vi "Meas Generate Freq List.vi"(2 "freq. id":i32, 3 "meas setup":T4={"swp cfg"={"N"=0, "R"=0, "f list"=[], "smpl delay"=0.0, "set delay"=0.0, "set delay np"=0.0, "meas root"=path "", "meas name"="", "meas a-index"=FALSE, "rnd sweep"=FALSE, "mode"=enum."Frequency", "swp mode"=enum."Linear", "avg"=0, "subrec"=0, "multi-freq"=FALSE}, "bridge"={"type"=enum."TWM client", "TWM"={"pipe name"="", "parameters"=[], "handle"=0, "fixed aper [s]"=0.0, "f-list [Hz]"=[], "discrete f-list"=FALSE, "unc mode"=enum."None", "unc mcc"=0, "unc first"=FALSE}, "last f"=0.0, "bias comp"={"bias type"=enum."dummy", "VISA"="", "Enable"=FALSE, "channel qu"=[], "channel Uinit"=[]}, "sim mode"=enum."Generic RLC network", "channel idns"=[], "sim phases"=1}, "src"={"type"=enum."Tektronix AFG3101C", "afg"={"VISA"="", "const"=0.0, "gen DC"=FALSE, "ext ref"=FALSE}, "cDAQ dds"={"device"="", "channels"=[], "mclk source"="", "mclk [Hz]"=0.0, "use ext mclk"=FALSE, "fs [Hz]"=0.0, "block [s]"=0.0, "buf [s]"=0.0, "task"="", "cmd queue"=refnum, "proc ref"=refnum, "smpl clock out"="/cDAQ3/PFI0", "export smpl clock"=FALSE, "DC ofs [V]"=[]}, "gain [V/A]"=1.0, "F5xxx session"={"VISA"="", "mode"=enum."AC voltage", "Earth on"=FALSE, "Ext ref lock"=FALSE}}, "results"=refnum} {"src"."cDAQ dds"."channels" min=0 step=1; "bridge"."TWM"."f-list [Hz]" format="%#_6p"; "swp cfg"."f list"."bias" format="%#_3p"; "swp cfg"."f list"."level" format="%#_3p"; "swp cfg"."f list"."fs [Hz]" format="%#_5p"; "swp cfg"."f list"."time [s]" format="%#_3p"; "swp cfg"."f list"."f/fs" format="%#_3p"; "swp cfg"."f list"."periods" format="%#_3f"; "swp cfg"."f list"."f [Hz]" format="%#_5p"}, 4 "config":T1={"swp type"=enum."Frequency", "freq sgl"=1000.0, "swp min"=0.0, "swp max"=0.0, "swp step"=0.0, "swp mode"=enum."Linear", "swp steps"=0, "round abs"=0.0, "round rel"=0.0, "f0 coherent"=FALSE, "min fs"=0.0, "min fs ratio"=0.0, "t int [s]"=0.0, "nper [-]"=0.0, "level sgl"=1000.0, "bias sgl"=1000.0, "single"=FALSE, "sweep"=FALSE, "custom"=FALSE, "swp list"=[], "skip mains"=FALSE, "N base"=0, "N max"=0, "N factor"=0.0, "N variable"=FALSE, "multi-freq"=FALSE} {"bias sgl" format="%#_6p"; "level sgl" format="%#_6p"; "freq sgl" format="%#_6p"}) -> (0 "freq lst":dbl[](array[numeric]) caption="Frequency list [Hz]" format="%#_6p", 1 "flist":T6[](array[typedef]) caption="Sweep list items" {"bias" format="%#_3p"; "level" format="%#_3p"; "fs [Hz]" format="%#_5p"; "time [s]" format="%#_3p"; "f/fs" format="%#_3p"; "periods" format="%#_3f"; "f [Hz]" format="%#_5p"})   [LabVIEW 2013]
doc: "Generate sweep list."
uses:
  Meas Freq Info.ctl
  meas session.ctl
  Meas Sweep Config.ctl
  meas_swp_mode.ctl
  meas_sweep_flist_mode.ctl
  bridge/Bridge Session.ctl
  bridge/Bridge Type.ctl
  drivers/TWM client/TWM Session.ctl
  drivers/TWM client/TWM parameters.ctl
  drivers/TWM client/Meas Proc QWTB Uncertainty Mode.ctl
  bridge/Bridge Bias Session.ctl
  bridge/Bridge Bias Type.ctl
  bridge/Bridge Sim Mode.ctl
  source/Source Session.ctl
  source/Source Type.ctl
  drivers/AFG3101C/AFG3101C Session.ctl
  drivers/cDAQ DDS/cDAQ DDS Session.ctl
  drivers/cDAQ DDS/cDAQ DDS Setup.ctl
  drivers/Fluke 5XXX/top_lev/F5xxx_session.ctl
  drivers/Fluke 5XXX/top_lev/F5xxx_output_mode.ctl
  Meas Results Ref.ctl
  Meas Results.ctl
  bridge/Bridge Frequency Readings Data.ctl
  drivers/TWM client/Meas Proc QWTB Spectrum Data.ctl
  drivers/TWM client/TWM Phase Info.ctl
  Meas Sweep List Generator Config.ctl
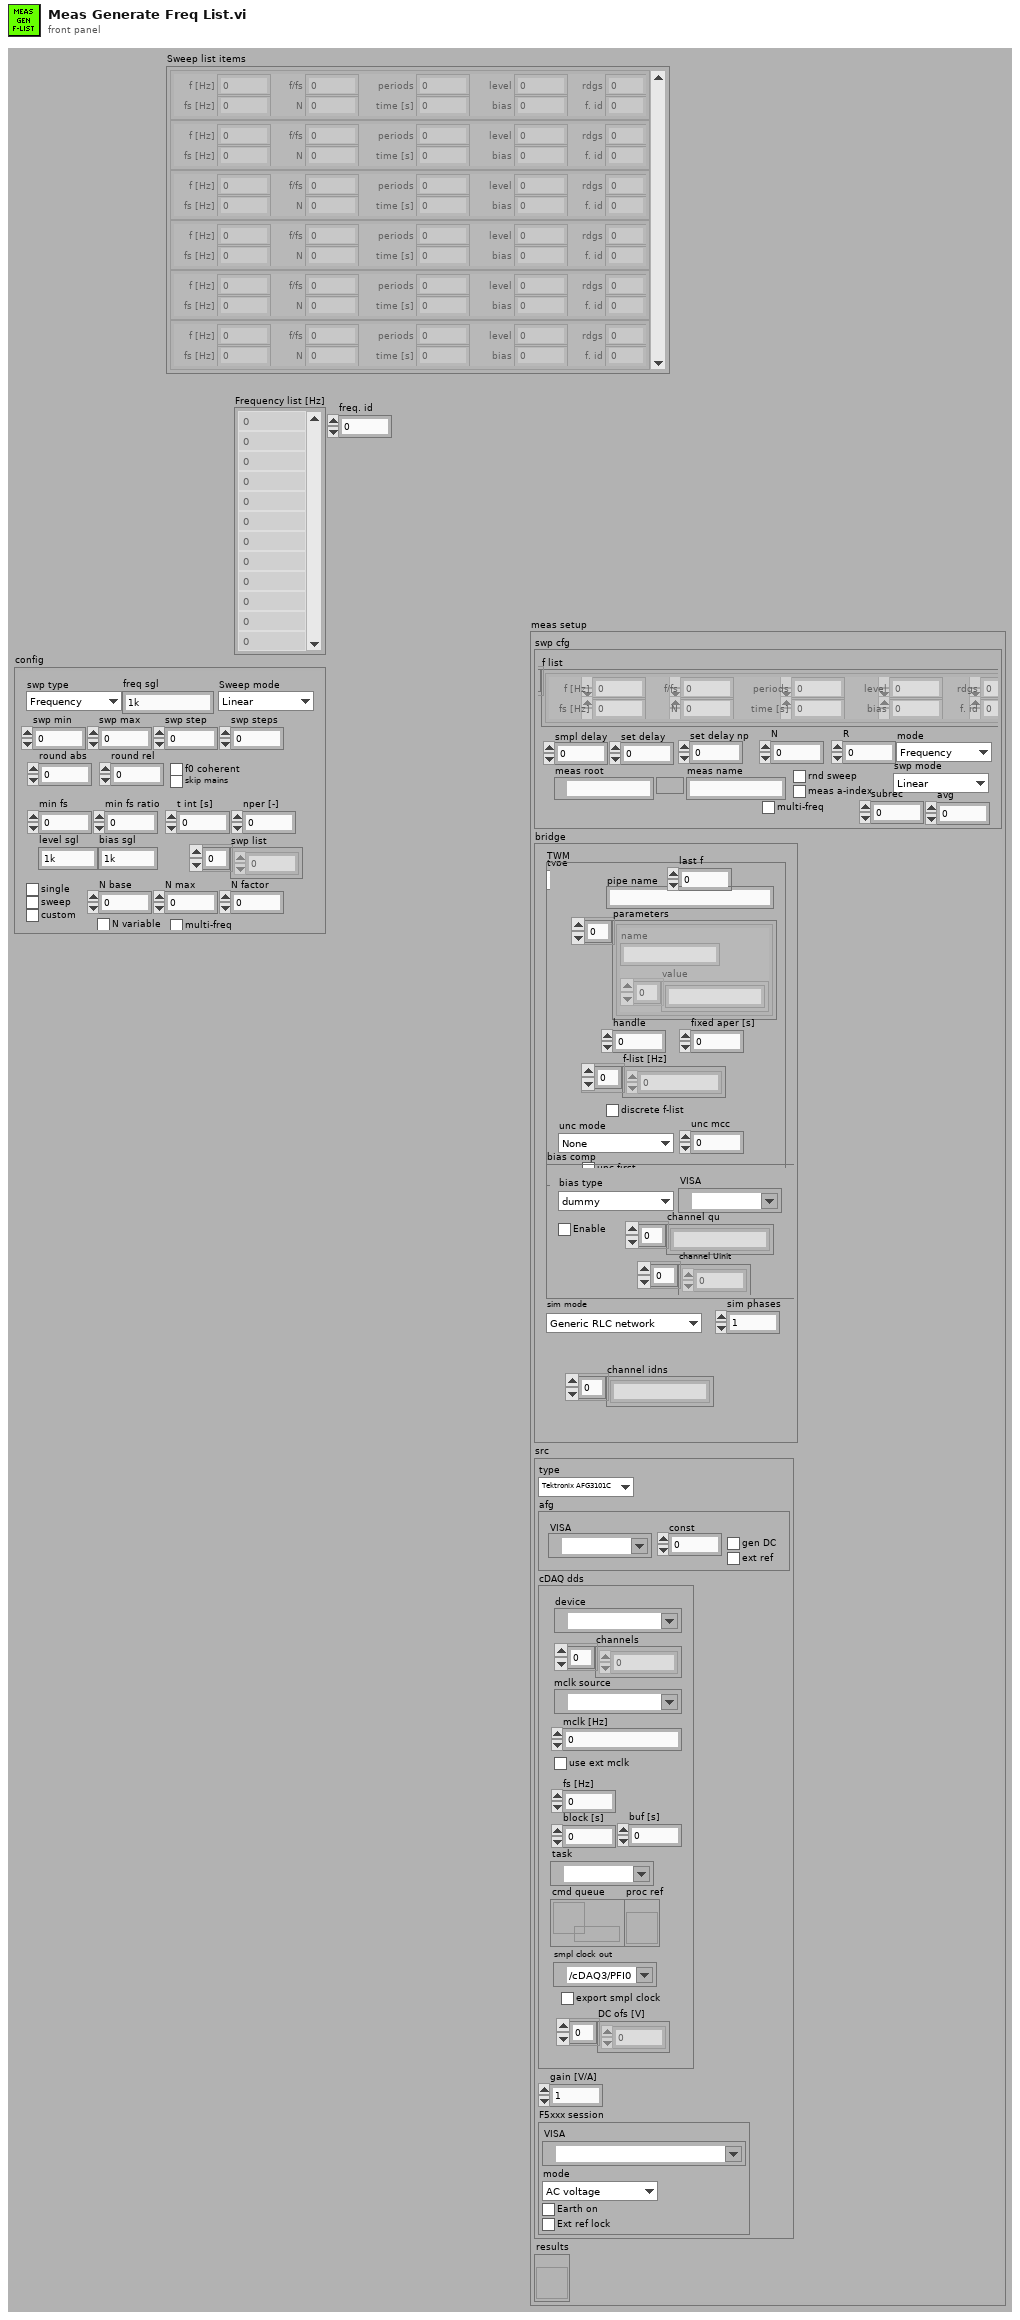
[diagram p1: front panel]
types:
  T1 = typedef "Meas Sweep List Generator Config.ctl" = cluster{"swp type":T2, "freq sgl":dbl, "swp min":dbl, "swp max":dbl, "swp step":dbl, "swp mode":T3, "swp steps":i32, "round abs":dbl, "round rel":dbl, "f0 coherent":bool, "min fs":dbl, "min fs ratio":dbl, "t int [s]":dbl, "nper [-]":dbl, "level sgl":dbl, "bias sgl":dbl, "single":bool, "sweep":bool, "custom":bool, "swp list":dbl[], "skip mains":bool, "N base":i32, "N max":i32, "N factor":dbl, "N variable":bool, "multi-freq":bool}
  T2 = typedef "meas_swp_mode.ctl" = enum16{"Frequency", "Level", "Bias"}
  T3 = typedef "meas_sweep_flist_mode.ctl" = enum16{"Linear", "Log10"}
  T4 = typedef "meas session.ctl" = cluster{"swp cfg":T5, "bridge":T7, "src":T15, "results":T21}
  T5 = typedef "Meas Sweep Config.ctl" = cluster{"N":i32, "R":i32, "f list":T6[], "smpl delay":dbl, "set delay":dbl, "set delay np":dbl, "meas root":path, "meas name":string, "meas a-index":bool, "rnd sweep":bool, "mode":T2, "swp mode":T3, "avg":i32, "subrec":i32, "multi-freq":bool}
  T6 = typedef "Meas Freq Info.ctl" = cluster{"f [Hz]":dbl, "periods":dbl, "f/fs":dbl, "time [s]":dbl, "fs [Hz]":dbl, "N":i32, "level":dbl, "bias":dbl, "rdgs":i32, "f. id":i32}
  T7 = typedef "Bridge Session.ctl" = cluster{"type":T8, "TWM":T9, "last f":dbl, "bias comp":T12, "sim mode":T14, "channel idns":string[], "sim phases":i32}
  T8 = typedef "Bridge Type.ctl" = enum16{"TWM client", "dummy"}
  T9 = typedef "TWM Session.ctl" = cluster{"pipe name":string, "parameters":T10[], "handle":i32, "fixed aper [s]":dbl, "f-list [Hz]":dbl[], "discrete f-list":bool, "unc mode":T11, "unc mcc":i32, "unc first":bool}
  T10 = typedef "TWM parameters.ctl" = cluster{"name":string, "value":string[]}
  T11 = typedef "Meas Proc QWTB Uncertainty Mode.ctl" = enum16{"None", "GUF", "Monte Carlo"}
  T12 = typedef "Bridge Bias Session.ctl" = cluster{"bias type":T13, "VISA":refnum<visa-resource-name>, "Enable":bool, "channel qu":string[], "channel Uinit":dbl[]}
  T13 = typedef "Bridge Bias Type.ctl" = enum16{"dummy", "CMI LiBbias V1.0"}
  T14 = typedef "Bridge Sim Mode.ctl" = enum16{"Generic RLC network", "Interchannel transfer"}
  T15 = typedef "Source Session.ctl" = cluster{"type":T16, "afg":T17, "cDAQ dds":T18, "gain [V/A]":dbl, "F5xxx session":T19}
  T16 = typedef "Source Type.ctl" = enum16{"Tektronix AFG3101C", "cDAQ DAC", "Fluke 5xxx", "Agilent 33120A", "dummy"}
  T17 = typedef "AFG3101C Session.ctl" = cluster{"VISA":refnum<visa-resource-name>, "const":dbl, "gen DC":bool, "ext ref":bool}
  T18 = typedef "cDAQ DDS Session.ctl" = cluster{"device":tag, "channels":i32[], "mclk source":tag, "mclk [Hz]":dbl, "use ext mclk":bool, "fs [Hz]":dbl, "block [s]":dbl, "buf [s]":dbl, "task":refnum<k21>, "cmd queue":refnum<queue>, "proc ref":refnum<vi>, "smpl clock out":tag, "export smpl clock":bool, "DC ofs [V]":dbl[]}
  T19 = typedef "F5xxx_session.ctl" = cluster{"VISA":refnum<visa-resource-name>, "mode":T20, "Earth on":bool, "Ext ref lock":bool}
  T20 = typedef "F5xxx_output_mode.ctl" = enum16{"AC voltage", "AC current"}
  T21 = typedef "Meas Results Ref.ctl" = refnum<vi>
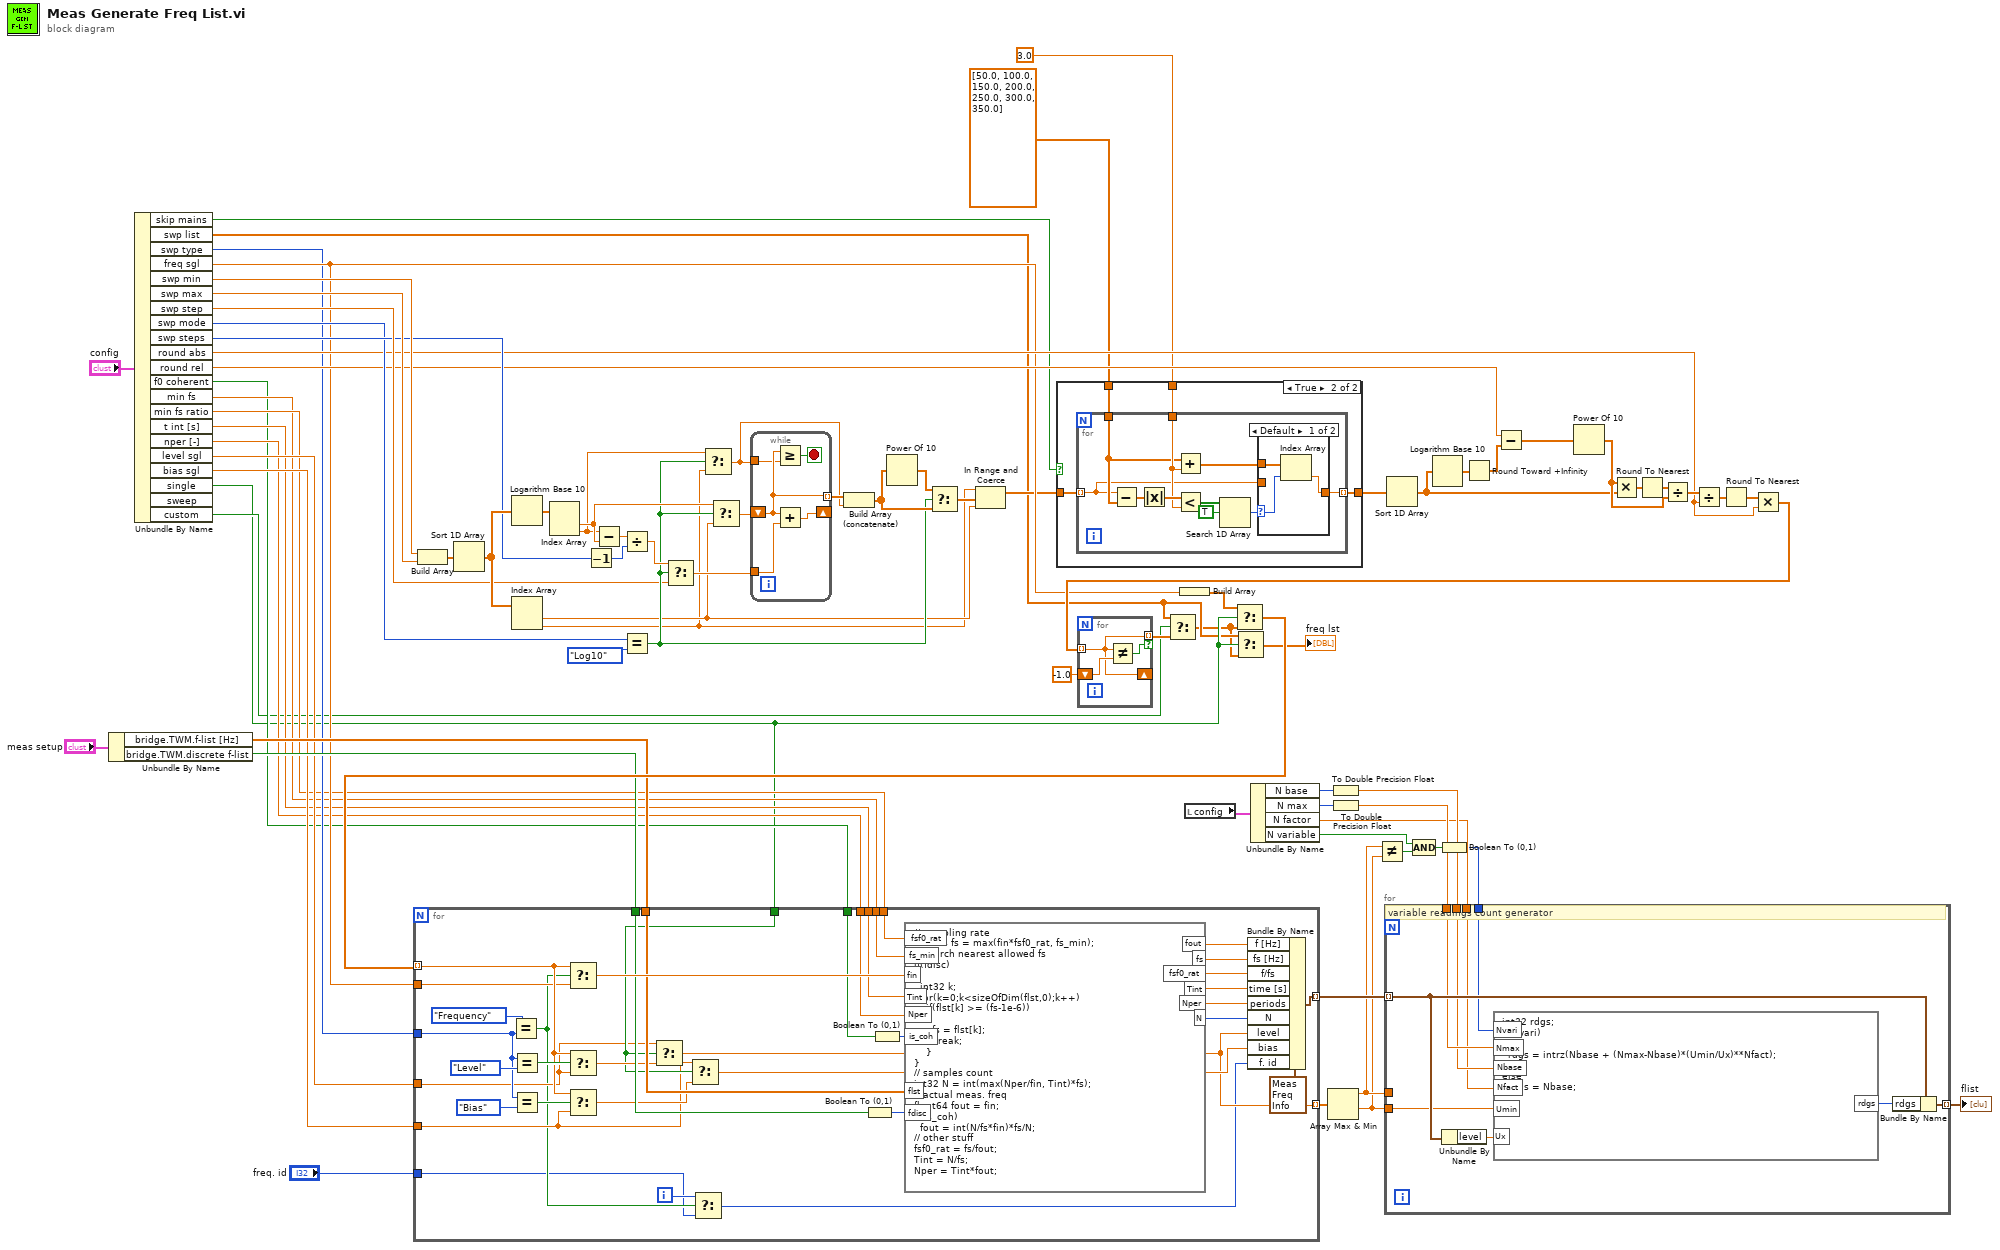
[diagram p0: block diagram]
diagram:
  n1 = Unbundle By Name("meas setup") -> ("bridge.TWM.f-list [Hz]"=w45:dbl[], "bridge.TWM.discrete f-list"=w46:bool)
  n2 = Unbundle By Name("config") -> ("skip mains"=w21:bool, "swp list"=w2:dbl[], "swp type"=w35:T2, "freq sgl"=w36:dbl, "swp min"=w43:dbl, "swp max"=w42:dbl, "swp step"=w41:dbl, "swp mode"=w39:T3, "swp steps"=w40:i32, "round abs"=w37:dbl, "round rel"=w38:dbl, "f0 coherent"=w28:bool, "min fs"=w31:dbl, "min fs ratio"=w32:dbl, "t int [s]"=w30:dbl, "nper [-]"=w29:dbl, "level sgl"=w34:dbl, "bias sgl"=w33:dbl, "single"=w4:bool, "custom"=w27:bool)  [unwired: 1 out]
  n3 = Build Array(w43, w42) -> (w80:dbl[])
  n4 = Sort 1D Array(array=w80) -> (sorted array=w79:dbl[])
  n5 = Logarithm Base 10(1:w79) -> (0:w78:dbl[])
  n6 = Index Array(array=w79) -> (element #1=w48:dbl, element #2=w47:dbl)  [unwired: 2 in]
  n7 = Index Array(array=w78) -> (element #1=w75:dbl, element #2=w73:dbl)  [unwired: 2 in]
  n8 = Decrement(x=w40) -> (x-1=w50:i32)
  n9 = Subtract(x=w73, y=w75) -> (x-y=w77:dbl)
  n10 = Divide(x=w77, y=w50) -> (x/y=w76:dbl)
  n11 = Equal?(x=w39, y=meas_sweep_flist_mode."Log10") -> (x = y?=w65:bool)
  n12 = Select(t=w76, s=w65, f=w41) -> (s? t:f=w74:dbl)
  n13 = Select(t=w73, s=w65, f=w47) -> (s? t:f=w68:dbl)
  n14 = Select(t=w75, s=w65, f=w48) -> (s? t:f=w71:dbl)
  n15 = while {
    tunnel: w74 -> [w85]
    tunnel: w68 -> [w82]
    shift-right: [w84] -> _
    shift-left: w71 -> [w83]
    tunnel: [w83] -> w72 mode=indexing
    stop <- w81 stop-if-true
    n16 = Greater Or Equal?(x=w83, y=w82) -> (x >= y?=w81:bool)
    n17 = Add(x=w83, y=w85) -> (x+y=w84:dbl)
  }
  n18 = Build Array (concatenate)(w72, w68) -> (w69:dbl[])
  n19 = Power Of 10(x=w69) -> (10^x=w70:dbl[])
  n20 = Select(t=w70, s=w65, f=w69) -> (s? t:f=w49:dbl[])
  n21 = In Range and Coerce(upper limit=w47, x=w49, lower limit=w48) -> (coerced(x)=w25:dbl[])  [unwired: 1 out]
  n22 = case shown="True" w21 {
    tunnel: w25 -> [w86 w90]
    tunnel: [w86 w89] -> w24
    tunnel: dbl[] [50.0, 100.0, 150.0, 200.0, 250.0, 300.0, 350.0] -> [_ w88]
    tunnel: 3.0 -> [_ w87]
    frame False {
    }
    frame True {
      n23 = for {
        tunnel: w90 -> [w92] mode=indexing
        tunnel: [w93] -> w89 mode=indexing
        tunnel: w88 -> [w97]
        tunnel: w87 -> [w98]
        n24 = Subtract(x=w92, y=w97) -> (x-y=w100:dbl[])
        n25 = Absolute Value(x=w100) -> (abs(x)=w99:dbl[])
        n26 = Add(x=w97, y=w98) -> (x+y=w91:dbl[])
        n27 = Less?(x=w99, y=w98) -> (x < y?=w96:bool[])
        n28 = Search 1D Array(1D array=w96, element=TRUE) -> (index of element=w94:i32)  [unwired: 1 in]
        n29 = case shown="Default" w94 {
          selector: w94 -> [w102 _]
          tunnel: [w101 w104] -> w93
          tunnel: w92 -> [_ w104]
          tunnel: w91 -> [w103 _]
          frame Default {
            n30 = Index Array(array=w103, index=w102) -> (element=w101:dbl)
          }
          frame -1 {
          }
        }
      }
    }
  }
  n31 = Build Array(w36) -> (w52:dbl[])
  n32 = local read "config"() -> (w19:T1)
  n33 = Unbundle By Name(w19) -> ("N base"=w16:i32, "N max"=w13:i32, "N factor"=w12:dbl, "N variable"=w7:bool)
  n34 = To Double Precision Float(number=w16) -> (double precision float=w15:dbl)
  n35 = To Double Precision Float(number=w13) -> (double precision float=w17:dbl)
  n36 = Sort 1D Array(array=w24) -> (sorted array=w58:dbl[])
  n37 = Logarithm Base 10(1:w58) -> (0:w64:dbl[])
  n38 = Round Toward +Infinity(x=w64) -> (ceil(x): smallest int >= x=w63:dbl[])
  n39 = Subtract(x=w38, y=w63) -> (x-y=w62:dbl[])
  n40 = Power Of 10(x=w62) -> (10^x=w59:dbl[])
  n41 = Multiply(x=w59, y=w58) -> (x*y=w61:dbl[])
  n42 = Round To Nearest(number=w61) -> (nearest integer value=w60:dbl[])
  n43 = Divide(x=w60, y=w59) -> (x/y=w57:dbl[])
  n44 = Divide(x=w57, y=w37) -> (x/y=w56:dbl[])
  n45 = Round To Nearest(number=w56) -> (nearest integer value=w55:dbl[])
  n46 = Multiply(x=w55, y=w37) -> (x*y=w54:dbl[])
  n47 = for {
    tunnel: w54 -> [w106] mode=indexing
    shift-right: [w106] -> _
    shift-left: -1.0 -> [w107]
    tunnel: [w106] -> w53 mode=indexing if=w105
    n48 = Not Equal?(x=w106, y=w107) -> (x != y?=w105:bool)
  }
  n49 = Select(t=w2, s=w27, f=w53) -> (s? t:f=w1:dbl[])
  n50 = Select(t=w52, s=w4, f=w1) -> (s? t:f=w51:dbl[])
  n51 = for {
    tunnel: w51 -> [w137] mode=indexing
    tunnel: [w143] -> w20 mode=indexing
    tunnel: w46 -> [w126]
    tunnel: w45 -> [w127]
    tunnel: w4 -> [w122]
    tunnel: w36 -> [w121]
    tunnel: w35 -> [w120]
    tunnel: w34 -> [w119]
    tunnel: w33 -> [w118]
    tunnel: w32 -> [w117]
    tunnel: w31 -> [w116]
    tunnel: w30 -> [w115]
    tunnel: w29 -> [w114]
    tunnel: w28 -> [w113]
    tunnel: [w112] -> w18 mode=indexing
    tunnel: "freq. id" -> [w108]
    i -> [w110]
    n52 = Equal?(x=meas_swp_mode."Frequency", y=w120) -> (x = y?=w111:bool)
    n53 = Equal?(x=w120, y=meas_swp_mode."Level") -> (x = y?=w140:bool)
    n54 = Equal?(x=w120, y=meas_swp_mode."Bias") -> (x = y?=w139:bool)
    n55 = Select(t=w137, s=w111, f=w121) -> (s? t:f=w136:dbl)
    n56 = Select(t=w137, s=w140, f=w119) -> (s? t:f=w125:dbl)
    n57 = Select(t=w137, s=w139, f=w118) -> (s? t:f=w124:dbl)
    n58 = Select(t=w119, s=w122, f=w125) -> (s? t:f=w112:dbl)
    n59 = Select(t=w118, s=w122, f=w124) -> (s? t:f=w123:dbl)
    n60 = Select(t=w110, s=w111, f=w108) -> (s? t:f=w109:i32)
    n61 = Boolean To (0,1)(Boolean=w126) -> (0, 1=w128:i16)
    n62 = Boolean To (0,1)(Boolean=w113) -> (0, 1=w135:i16)
    n63 = formula code="// sampling rate\nfloat64 fs = max(fin*fsf0_rat, fs_min);\n// search nearest allowed fs\nif(fdisc)\n{\n  int32 k;\n  for(k=0;k<sizeOfDim(flst,0);k++)\n    if(flst[k] >= (fs-1e-6))\n    {\n      fs = flst[k];\n      break;\n    }\n}\n// samples count\nint32 N = int(max(Nper/fin, Tint)*fs);\n// actual meas. freq\nfloat64 fout = fin;\nif(is_coh)\n  fout = int(N/fs*fin)*fs/N;\n// other stuff\nfsf0_rat = fs/fout;\nTint = N/fs;\nNper = Tint*fout;"("fsf0_rat"=w117, "fs_min"=w116, "Tint"=w115, "Nper"=w114, "fin"=w136, "is_coh"=w135, "flst"=w127, "fdisc"=w128) -> ("fout"=w134:dbl, "fs"=w133:dbl, "Tint"=w131:dbl, "Nper"=w130:dbl, "fsf0_rat"=w132:dbl, "N"=w129:i32)
    n64 = Bundle By Name(cluster=T6 {"f [Hz]"=0.0, "periods"=0.0, "f/fs"=0.0, "time [s]"=0.0, "fs [Hz]"=0.0, "N"=0, "level"=0.0, "bias"=0.0, "rdgs"=0, "f. id"=0} ("Cluster"), "f [Hz]"=w134, "fs [Hz]"=w133, "f/fs"=w132, "time [s]"=w131, "periods"=w130, "N"=w129, "level"=w112, "bias"=w123, "f. id"=w109) -> (w143:T6)
  }
  n65 = Select(t=w2, s=w4, f=w1) -> (s? t:f=→"freq lst":dbl[])
  n66 = Array Max & Min(array=w18) -> (max value=w10:dbl, min value=w9:dbl)  [unwired: 2 out]
  n67 = Not Equal?(x=w10, y=w9) -> (x != y?=w8:bool)
  n68 = Compound Arithmetic op=AND(w7, w8) -> (w6:bool)
  n69 = Boolean To (0,1)(Boolean=w6) -> (0, 1=w11:i16)
  n70 = for {
    tunnel: w20 -> [w153] mode=indexing
    tunnel: w9 -> [w151]
    tunnel: w10 -> [_]
    tunnel: w17 -> [w150]
    tunnel: w15 -> [w149]
    tunnel: [w152] -> w14 mode=indexing
    tunnel: w12 -> [w148]
    tunnel: w11 -> [w146]
    # "variable readings count generator"
    n71 = Unbundle By Name(w153) -> ("level"=w147:dbl)
    n72 = formula code="int32 rdgs;\nif(Nvari)\n{\n  rdgs = intrz(Nbase + (Nmax-Nbase)*(Umin/Ux)**Nfact);\n}\nelse\n  rdgs = Nbase;"("Nmax"=w150, "Nbase"=w149, "Nfact"=w148, "Umin"=w151, "Ux"=w147, "Nvari"=w146) -> ("rdgs"=w145:i32)
    n73 = Bundle By Name(cluster=w153, "rdgs"=w145) -> (w152:T6)
  }
  "flist" <- w14
